vi "Instructions to Add Preferences Editor Support.vi"   [LabVIEW 2020, in "Rename As Application UI.lvlib" / "Configuration.lvlib"]
doc: "See Block diagram for VI Tree for the Configuration Library and for instructions on how to add DCFG Framework support to other modules.\n_____\nBased on DCFG Project Template 1.0.0.21.\n____\nPeloton Config 1.0.0.2\nCopyright (c) 2022, Peloton"
uses:
  Configuration.lvlib
  Configuration--cluster.ctl
  <vilib>/Peloton/Peloton Config/Libraries/DCFG Framework/Peloton_DCFG Framework.lvlib
panel:
  # "See Block diagram for VI Tree for instructions on how to add DCFG Framework support to other modules."
types:
  T1 = typedef "Rename As Application UI.lvlib/Configuration.lvlib/Configuration--cluster.ctl" = cluster{"Logging Path":path}
  T2 = typedef "Peloton_DCFG Framework.lvlib/Broadcast Events--cluster.ctl" = cluster{"Module Did Init":refnum<user-event>, "Status Updated":refnum<user-event>, "Error Reported":refnum<user-event>, "Module Did Stop":refnum<user-event>, "Update Module Execution Status":refnum<user-event>, "View Changed":refnum<user-event>, "Configuration Updated":refnum<user-event>, "Page Error Received":refnum<user-event>, "Page List Updated":refnum<user-event>, "Defaults Applied":refnum<user-event>, "Main Window Closed":refnum<user-event>}
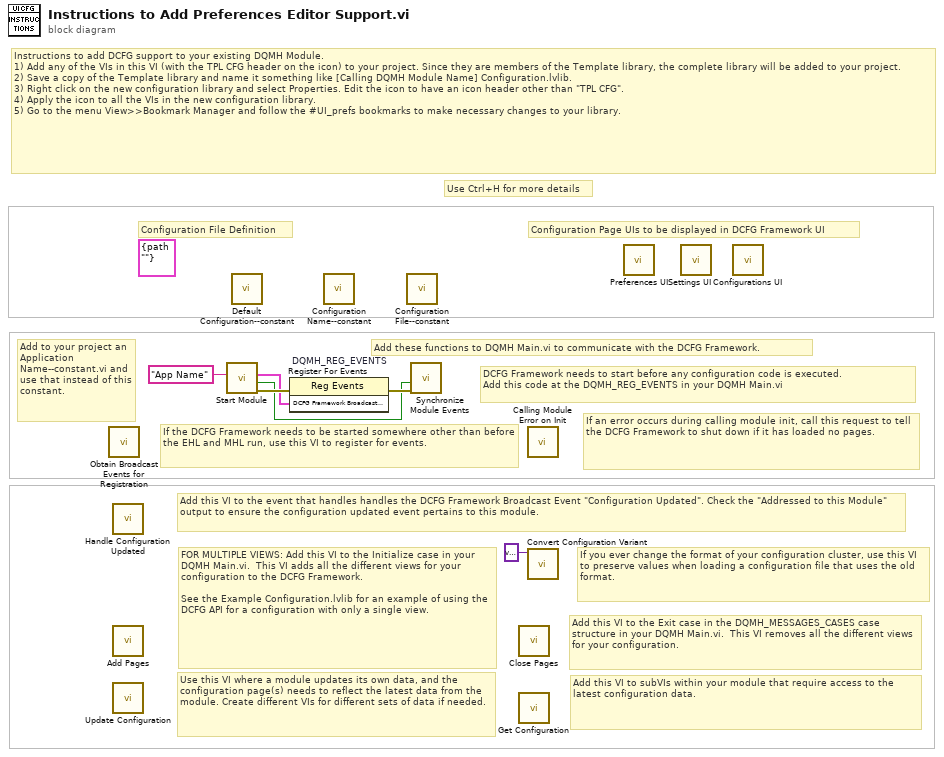
[diagram p0: block diagram]
diagram:
  (unwired) T1 {"Logging Path"=path ""} ("Default Configuration")
  # "Add to your project an Application Name--constant.vi and use that instead of this constant."
  # "If you ever change the format of your configuration cluster, use this VI to preserve values when loading a configuration file that uses the old format."
  # "If an error occurs during calling module init, call this request to tell the DCFG Framework to shut down if it has loaded no pages."
  # "Add this VI to subVIs within your module that require access to the latest configuration data."
  # "Configuration Page UIs to be displayed in DCFG Framework UI"
  # "Use Ctrl+H for more details"
  # "Use this VI where a module updates its own data, and the configuration page(s) needs to reflect the latest data from the module. Create different VIs for different sets of data if needed."
  # "Add this VI to the Exit case in the DQMH_MESSAGES_CASES case structure in your DQMH Main.vi.  This VI removes all the different views for your configuration."
  # "FOR MULTIPLE VIEWS: Add this VI to the Initialize case in your DQMH Main.vi.  This VI adds all the different views for your configuration to the DCFG Framework.\n\nSee the Example Configuration.lvlib for an example of using the DCFG API for a configuration with only a single view."
  # "Add this VI to the event that handles handles the DCFG Framework Broadcast Event \"Configuration Updated\". Check the \"Addressed to this Module\" output to ensure the configuration updated event pertains to this module."
  # "If the DCFG Framework needs to be started somewhere other than before the EHL and MHL run, use this VI to register for events."
  # "DCFG Framework needs to start before any configuration code is executed.\nAdd this code at the DQMH_REG_EVENTS in your DQMH Main.vi"
  # "Add these functions to DQMH Main.vi to communicate with the DCFG Framework."
  # "Configuration File Definition"
  # "Instructions to add DCFG support to your existing DQMH Module.\n1) Add any of the VIs in this VI (with the TPL CFG header on the icon) to your project. Since they are members of the Template library, the complete library will be added to your project.\n2) Save a copy of the Template library and name it something like [Calling DQMH Module Name] Configuration.lvlib.\n3) Right click on the new configuration library and select Properties. Edit the icon to have an icon header other than \"TPL CFG\".\n4) Apply the icon to all the VIs in the new configuration library.\n5) Go to the menu View>>Bookmark Manager and follow the #UI_prefs bookmarks to make necessary changes to your library."
  n1 = call <vilib>:"Obtain Broadcast Events for Registration.vi"() -> ()  [unwired: 9 in, 3 out]
  n2 = call "Handle Configuration Updated.vi"() -> ()  [unwired: 9 in, 3 out]
  n3 = call "Add Pages.vi"() -> ()  [unwired: 10 in, 2 out]
  n4 = call "Update Configuration.vi"() -> ()  [unwired: 11 in, 1 out]
  n5 = call <vilib>:"Start Module.vi"("Application Name"="App Name") -> ("error out"=w6:errorcluster, "Wait for Event Sync?"=w3:bool, "DCFG Framework Broadcast Events"=w5:T2)  [unwired: 7 in, 1 out]
  n6 = call "Default Configuration--constant.vi"() -> ()  [unwired: 11 in, 1 out]
  n7 = register-events "DQMH_REG_EVENTS"(error in=w6, w5) -> (error out=w4:errorcluster)  [unwired: 1 in, 1 out]
  n8 = call "Configuration Name--constant.vi"() -> ()  [unwired: 11 in, 1 out]
  n9 = call "Configuration File--constant.vi"() -> ()  [unwired: 11 in, 1 out]
  n10 = call <vilib>:"Synchronize Module Events.vi"("error in (no error)"=w4, "Wait for Event Sync?"=w3) -> ()  [unwired: 9 in, 1 out]
  n11 = call "Close Pages.vi"() -> ()  [unwired: 10 in, 2 out]
  n12 = call "Get Configuration.vi"() -> ()  [unwired: 11 in, 1 out]
  n13 = call <vilib>:"Calling Module Error on Init.vi"() -> ()  [unwired: 11 in, 1 out]
  n14 = call "Convert Configuration Variant.vi"("Current Configuration"=variant) -> ()  [unwired: 8 in, 3 out]
  n15 = call "Preferences UI.vi"() -> ()  [unwired: 12 in]
  n16 = call "Settings UI.vi"() -> ()  [unwired: 12 in]
  n17 = call "Configurations UI.vi"() -> ()  [unwired: 12 in]
